vi "selectSubVI.vi"(1 "ItemTag":string) -> (0 "MainStateQueue":T1)   [LabVIEW 2010]
uses:
  MainStateQueueType.ctl
  MainStates.ctl
  MainGlobalConstants.vi
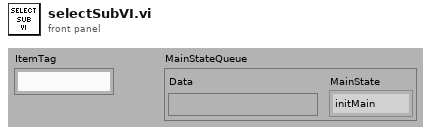
[diagram p1: front panel]
types:
  T1 = typedef "MainStateQueueType.ctl" = cluster{"Data":variant, "MainState":T2}
  T2 = typedef "MainStates.ctl" = enum16{"initMain", "insertSubVI", "startSubVI", "stopSubVI", "Exit", "ERROR", "idle"}
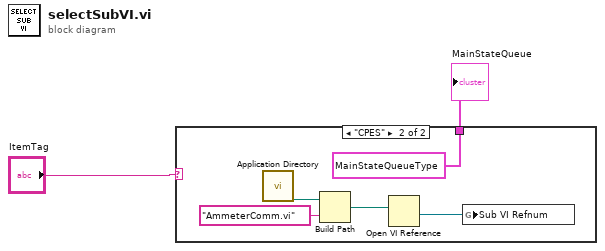
[diagram p0: block diagram]
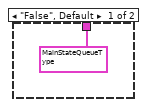
[diagram p2: hidden frame]
diagram:
  n1 = case shown="\"CPES\"" "ItemTag" {
    tunnel: [T1 {"Data"=variant, "MainState"=enum."idle"} ("MainStateQueue") T1 {"Data"=variant, "MainState"=enum."insertSubVI"} ("MainStateQueue")] -> w2
    frame "False", Default {
    }
    frame "CPES" {
      n2 = call <vilib>:"Application Directory.vi"() -> ("Application Directory"=w8:path)
      n3 = Build Path(base path=w8, name or relative path="AmmeterComm.vi") -> (appended path=w6:path)
      n4 = Open VI Reference(vi path=w6) -> (vi reference=w5:refnum<vi>)  [unwired: 5 in, 1 out]
      n5 = global write "MainGlobalConstants.vi" "Sub VI Refnum"(w5) -> ()
    }
  }
  "MainStateQueue" <- w2
